vi "_getDataPluginUrlType.vi"(10 "DataPlugin Index":i32, 11 "DataPlugin information":T1[](array[typedef])) -> (2 "type":string, 3 "Url":string)   [LabVIEW 2017]
uses:
  <vilib>/Platform/storage/utility/DataPluginSynchronization/_DataPluginInfo.ctl
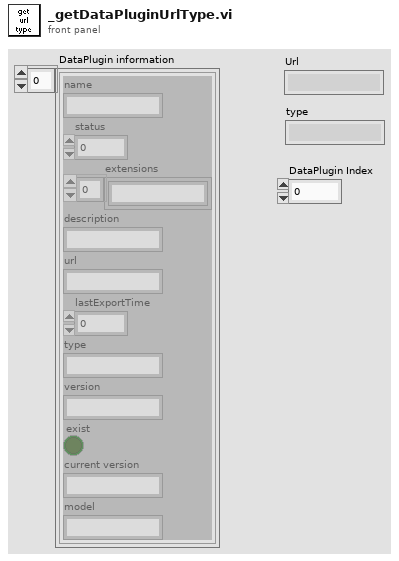
[diagram p1: front panel]
types:
  T1 = typedef "_DataPluginInfo.ctl" = cluster{"name":string, "status":u32, "extensions":string[], "description":string, "url":string, "lastExportTime":i64, "type":string, "version":string, "exist":bool, "current version":string, "model":string}
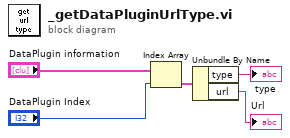
[diagram p0: block diagram]
diagram:
  n1 = Index Array(array="DataPlugin information", index="DataPlugin Index") -> (element=w3:T1)
  n2 = Unbundle By Name(w3) -> ("type"=→"type":string, "url"=→"Url":string)
